vi "PartyMode.vi"(10 "Reset":bool, 11 "Driver A":bool) -> ()   [LabVIEW 2018]
uses:
  Actions.ctl
  Framework/Robot Global Data.vi
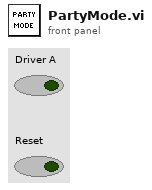
[diagram p1: front panel]
types:
  T1 = typedef "Actions.ctl" = enum16{"Default", "Hatch Triggered", "Lost Vision", "Auto Aiming", "Party Mode", "Has Hatch", "Brownout", "Height Setpoint"}
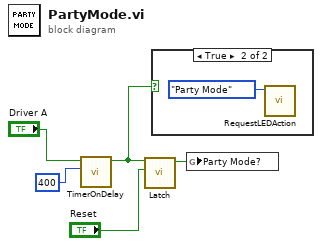
[diagram p0: block diagram]
diagram:
  n1 = call "TimerOnDelay.vi"("Time Limit"=u32 400, "Input"="Driver A") -> ("Output"=w1:bool)  [unwired: 9 in]
  n2 = call "Latch.vi"("Reset"="Reset", "Input"=w1) -> ("Output"=w3:bool)  [unwired: 9 in]
  n3 = case shown="True" w1 {
    frame False {
    }
    frame True {
      n4 = call "RequestLEDAction.vi"("Action"=Actions."Party Mode") -> ()  [unwired: 11 in]
    }
  }
  n5 = global write "Robot Global Data.vi" "Party Mode?"(w3) -> ()
